vi "FPGA Main.vi"() -> ()   [LabVIEW 2014]
uses:
  <vilib>/rvi/Emulation/niFpgaGetClockAttributes.vi
  <vilib>/rvi/Emulation/niFpgaSctlEmulationGetInTimedLoop.vi
  <vilib>/rvi/Emulation/niFpgaEmulationReportErrorSimple.vi
  <vilib>/rvi/interface/RandomDataEmulation/niFpgaRandomDataHandleErrors.vi
  <vilib>/rvi/eio/common/nirviEmuTemplateMethod_errors.vi
  <vilib>/rvi/Emulation/niFpgaCriticalErrorInLSC.vi
  <vilib>/rvi/Emulation/niFpgaProcessEmulError.vi
  <vilib>/rvi/Emulation/niFpgaEmulationIsFPGAContextNoSignature.vi
  <vilib>/rvi/errors/niFpgaSetErrorForExecOnDevCompSimple.vi
  <vilib>/rvi/eio/common/nirviEmuReportErrorAndStop.vi
  <vilib>/rvi/DataTransferAndStorage/Container/Common/niFpgaContainerGetUniqueNameForEmu.vi
  <vilib>/rvi/FIFO/Fifo_Resource/nirvififoEmulationSetSize.vi
  <vilib>/rvi/FIFO/Fifo_Resource/nirviFifoEmulationQueueMgr.vi
  <instcachedir>/0/nirviFifoEmulationQueueMgr_E5CAEC123FF24DC58D834DCA3CDAA9B5.lvgen/nirviFifoEmulationQueueMgr_E5CAEC123FF24DC58D834DCA3CDAA9B5_002.vi
  <vilib>/rvi/FIFO/Fifo_Resource/nirvififoEmulationCreateLock.vi
  <vilib>/rvi/FIFO/Fifo_Resource/nirvififoEmulationObtainLock.vi
  <vilib>/rvi/FIFO/Fifo_Resource/nirvififoEmulationReleaseLock.vi
  <vilib>/rvi/occurrence/nirviWaitOnOccurrenceBase.vi
  <vilib>/rvi/errors/nirviReportUnexpectedCaseInternalError.vi
  <vilib>/rvi/errors/nirviReportUnexpectedCaseInternalError (U32).vi
  Sub VIs/MIDI/Controls/Stop.vi
  <vilib>/rvi/DataTransferAndStorage/Container/XNode/niFpgaContainer.xnode
  <vilib>/rvi/interface/RandomDataEmulation/nirviRandomDataFpgaReadWriteTemplate.vi
  <vilib>/eio/EIONode/EIONode.xnode
  <vilib>/rvi/FIFO/Fifo_Resource/nirvififoEmulationRead.vi
panel:
  out "Read: Char":u8
  out "Read: New Data":bool
  in  "FPGA STOP":bool
  out "Actual Period (tics)":u32
  in  "Count(Ticks)":u32=907
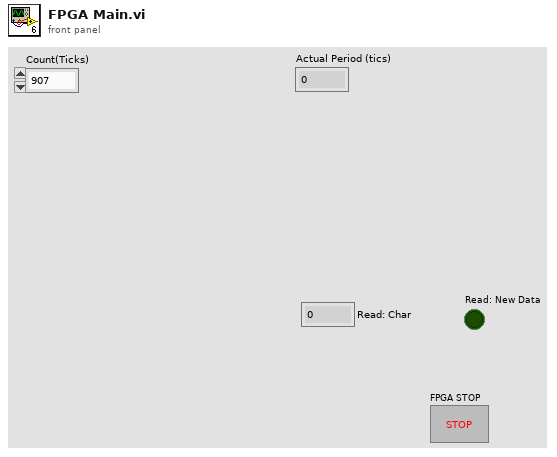
[diagram p1: front panel]
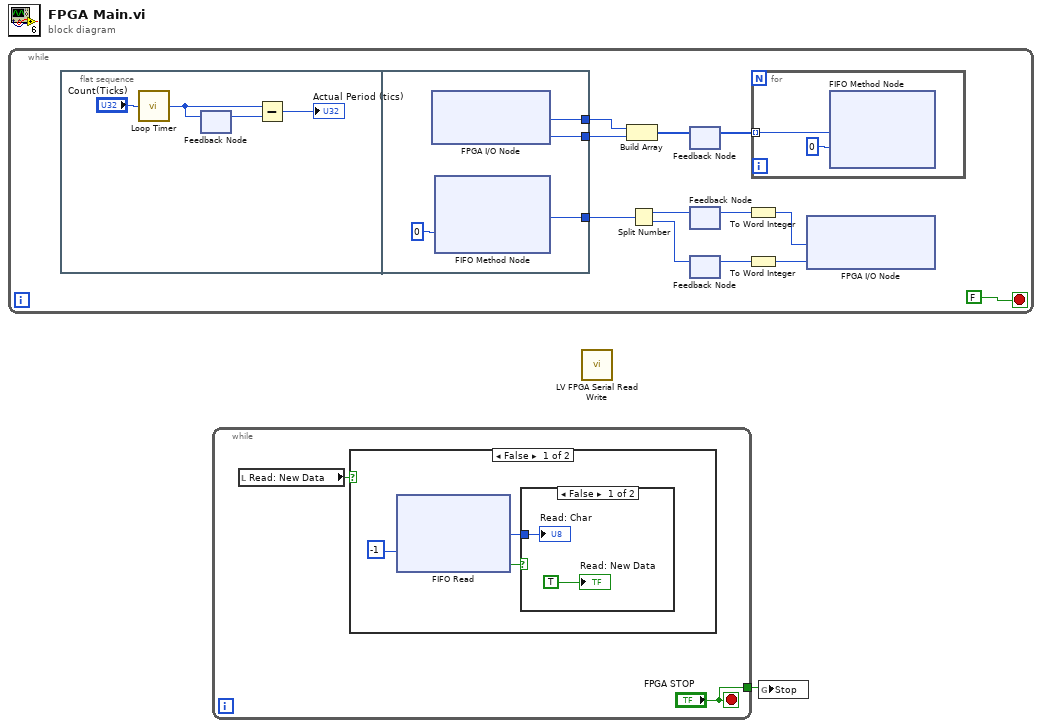
[diagram p0: block diagram]
diagram:
  n1 = while {
    stop <- FALSE stop-if-true
    n2 = flat-sequence {
      tunnel: [w23] -> w10
      tunnel: [w22] -> w8
      tunnel: [w21] -> w9
      frame #0 {
        n3 = call "Loop Timer"("Count(Ticks)"="Count(Ticks)") -> ("Tick Count(Ticks)"=w18:u32)
        n4 = feedback-in #1(w18) -> ()
        n5 = feedback #1() -> (w17:u32)  [unwired: 1 in]
        n6 = Subtract(x=w18, y=w17) -> (x-y=→"Actual Period (tics)":u32)
      }
      frame #1 {
        n7 = xnode "FPGA I/O Node"() -> ("AudioIn/Left"=w23:i16, "AudioIn/Right"=w21:i16)  [unwired: 2 in, 2 out]
        n8 = xnode ("FIFO Method Node")("Timeout"=0) -> ("Element"=w22:u32)  [unwired: 1 in, 2 out]
      }
    }
    n9 = Build Array(w10, w9) -> (w12:i16[])
    n10 = Split Number(x=w8) -> (hi(x)=w7:u16, lo(x)=w6:u16)
    n11 = feedback-in #2(w12) -> ()
    n12 = feedback #2() -> (w11:i16[])  [unwired: 1 in]
    n13 = feedback #3() -> (w2:u16)  [unwired: 1 in]
    n14 = feedback-in #3(w7) -> ()
    n15 = feedback #4() -> (w3:u16)  [unwired: 1 in]
    n16 = feedback-in #4(w6) -> ()
    n17 = To Word Integer(number=w2) -> (16bit integer=w5:i16)
    n18 = To Word Integer(number=w3) -> (16bit integer=w4:i16)
    n19 = for {
      tunnel: w11 -> [w15] mode=indexing
      n20 = xnode ("FIFO Method Node")("Element"=w15, "Timeout"=0) -> ()  [unwired: 1 in, 2 out]
    }
    n21 = xnode "FPGA I/O Node"("AudioOut/Left"=w5, "AudioOut/Right"=w4) -> ()  [unwired: 2 in, 2 out]
  }
  n22 = while {
    tunnel: ["FPGA STOP"] -> w1
    stop <- "FPGA STOP" stop-if-true
    n23 = local read "Read: New Data"() -> (w25:bool)
    n24 = case shown="False" w25 {
      frame False {
        n25 = xnode ("FIFO Read")("Timeout"=-1) -> ("Element"=w26:u8, "Timed Out?"=w27:bool)  [unwired: 1 in, 1 out]
        n26 = case shown="False" w27 {
          tunnel: w26 -> [w30 _]
          frame False {
            "Read: Char" <- w30
            "Read: New Data" <- TRUE ("Read: New Data")
          }
          frame True {
          }
        }
      }
      frame True {
      }
    }
  }
  n27 = call "LV FPGA Serial Read Write.vi"() -> ()  [unwired: 7 in, 9 out]
  n28 = global write "Stop.vi" "Stop"(w1) -> ()
